vi "OnOff Write.vi"(8 "error in":errorcluster, 10 "OnOff STS":i32, 11 "Chiller in":refnum<class "Chiller.lvclass">) -> (0 "error out":errorcluster, 3 "Chiller out":refnum<class "Chiller.lvclass">)   [LabVIEW 2023, in "Chiller.lvclass"]
uses:
  Chiller.lvclass
  Chiller.lvclass/Chiller.ctl
  Low Level Capabilities/OnOff/OnOff.lvclass
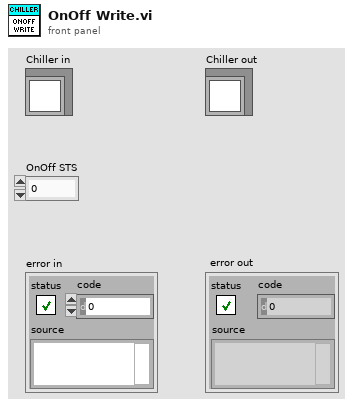
[diagram p1: front panel]
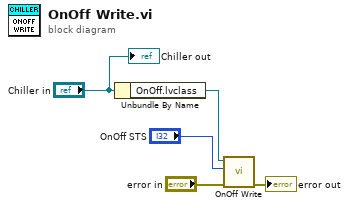
[diagram p0: block diagram]
diagram:
  n1 = Unbundle By Name("Chiller in") -> ("OnOff.lvclass"=w2:refnum<class "OnOff.lvclass">)
  n2 = call-dynamic "OnOff Write.vi"("error in"="error in", "OnOff STS"="OnOff STS", "OnOff in"=w2) -> ("error out"=→"error out":errorcluster)  [unwired: 7 in, 1 out]
  "Chiller out" <- "Chiller in"
